vi "lianjieStr.vi"(10 "data":string, 11 "area_name":string) -> (3 "连接后字符串":string)   [LabVIEW 2014, in "cyy.lvlib"]
uses:
  cyy.lvlib
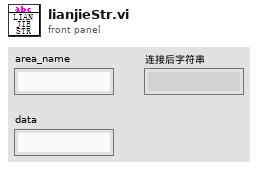
[diagram p1: front panel]
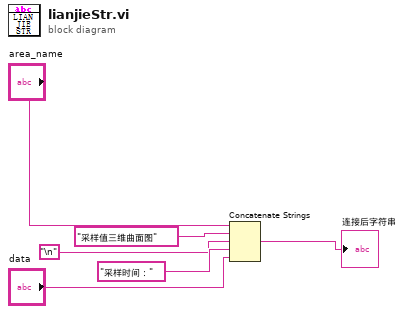
[diagram p0: block diagram]
diagram:
  n1 = Concatenate Strings("area_name", "采样值三维曲面图", "\n", "采样时间：", "data") -> (→"连接后字符串":string)
